vi "Get Charact By Standard Setting.vi"(11 "error in (no error)":errorcluster) -> (4 "Charact By Standard?":bool, 15 "error out":errorcluster)   [LabVIEW 2023, in "RFCalAndFixtureCharact.Common.lvlib"]
uses:
  RFCalAndFixtureCharact.Common.lvlib
  Data Cache/Settings Dictionary/Setting Keys.vi
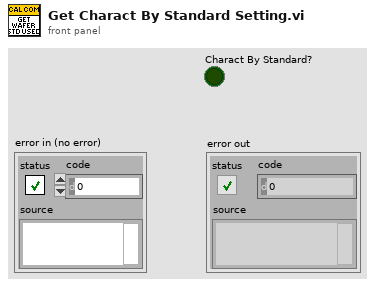
[diagram p1: front panel]
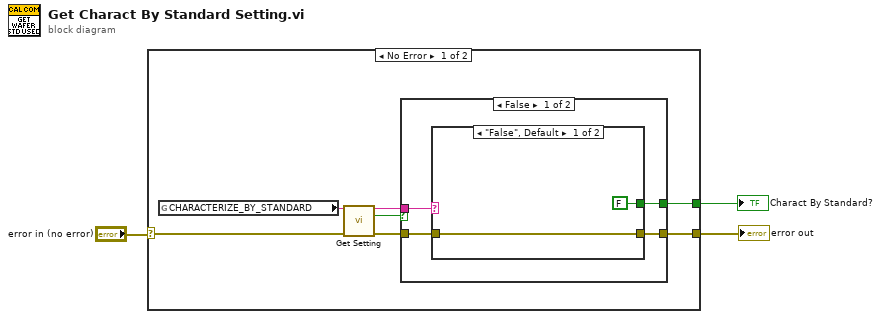
[diagram p0: block diagram]
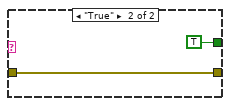
[diagram p2: hidden frame]
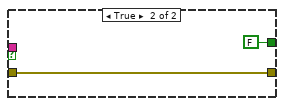
[diagram p3: hidden frame]
diagram:
  n1 = case shown="No Error" "error in (no error)" {
    selector: "error in (no error)" -> [w7 w21]
    tunnel: [w10 w21] -> w2
    tunnel: [w9 _] -> w1
    frame No Error {
      n2 = global read "Setting Keys.vi" "CHARACTERIZE_BY_STANDARD"() -> (w8:string)
      n3 = call "Get Setting.vi"("Setting name"=w8, "error in (no error)"=w7) -> ("Setting value out"=w4:string, "Setting empty or not found?"=w5:bool, "error out"=w6:errorcluster)  [unwired: 11 in]
      n4 = case shown="False" w5 {
        tunnel: [w13 w20] -> w10
        tunnel: w6 -> [w12 w20]
        tunnel: w4 -> [w14 _]
        tunnel: [w11 FALSE] -> w9
        frame False {
          n5 = case shown="\"False\", Default" w14 {
            tunnel: [w16 w18] -> w13
            tunnel: w12 -> [w16 w18]
            tunnel: [FALSE TRUE] -> w11
            frame "False", Default {
            }
            frame "True" {
            }
          }
        }
        frame True {
        }
      }
    }
    frame Error {
    }
  }
  "error out" <- w2
  "Charact By Standard?" <- w1
